vi "LVPortConvertObjectMapDataValueToVartiant.vi"(9 "Allow Variant Values (f)":bool, 10 "MatlabDataBundle":T1, 11 "Data Value":variant) -> (3 "Value":variant)   [LabVIEW 2017]
uses:
  LVPortObjectMapNamepathData.ctl
  LVPortObjectMapDataTypeEnum.ctl
  LVPortObjectMapContainerTypeEnum.ctl
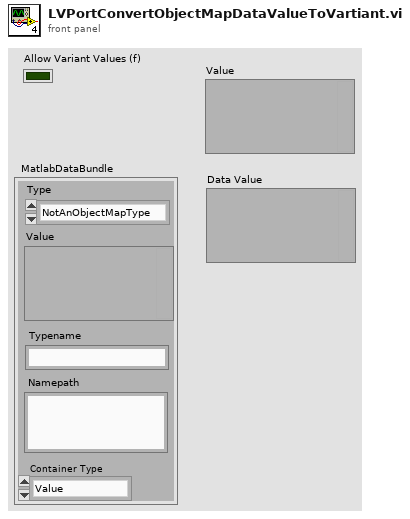
[diagram p1: front panel]
types:
  T1 = typedef "LVPortObjectMapNamepathData.ctl" = cluster{"Type":T2, "Value":variant, "Namepath":string, "Typename":string, "Container Type":T3}
  T2 = typedef "LVPortObjectMapDataTypeEnum.ctl" = enum16{"NotAnObjectMapType", "Real", "Complex", "String", "Boolean"}
  T3 = typedef "LVPortObjectMapContainerTypeEnum.ctl" = enum16{"Value", "Array", "Waveform"}
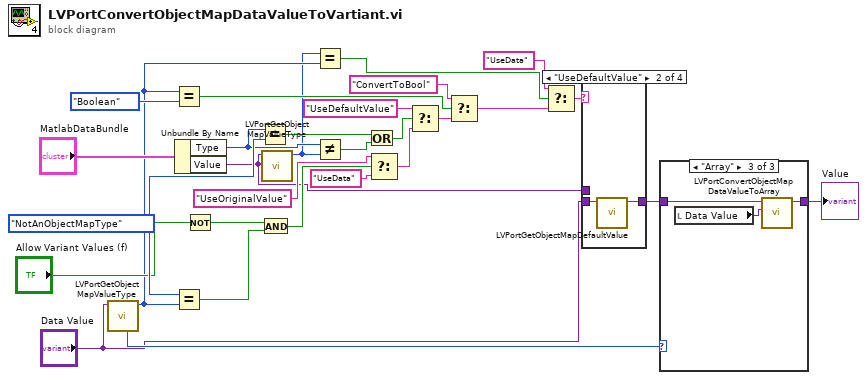
[diagram p0: block diagram]
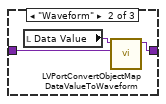
[diagram p3: hidden frame]
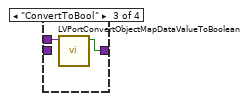
[diagram p5: hidden frame]
diagram:
  w20 = LVPortObjectMapDataTypeEnum."NotAnObjectMapType" ("MatlabType")
  n1 = call "LVPortGetObjectMapValueType.vi"("Value"="Data Value") -> ("ObjectMapType"=w10:T2, "Container Type (Labview Value type)"=w9:T3)  [unwired: 6 in, 3 out]
  n2 = Equal?(x=w10, y=LVPortObjectMapDataTypeEnum."Boolean" ("MatlabType")) -> (x = y?=w25:bool)
  n3 = Equal?(x=w20, y=w10) -> (x = y?=w17:bool)
  n4 = Unbundle By Name("MatlabDataBundle") -> ("Type"=w7:T2, "Value"=w4:variant)
  n5 = Not(x="Allow Variant Values (f)") -> (.not. x?=w19:bool)
  n6 = Equal?(x=w7, y=w20) -> (x = y?=w21:bool)
  n7 = And(x=w19, y=w17) -> (x .and. y?=w16:bool)
  n8 = call "LVPortGetObjectMapValueType.vi"("Value"=w4) -> ("ObjectMapType"=w1:T2)  [unwired: 6 in, 4 out]
  n9 = Equal?(x=w1, y=w10) -> (x = y?=w27:bool)
  n10 = Not Equal?(x=w7, y=w1) -> (x != y?=w5:bool)
  n11 = Or(x=w21, y=w5) -> (x .or. y?=w6:bool)
  n12 = Select(t="UseOriginalValue", s=w16, f="UseData") -> (s? t:f=w14:string)
  n13 = Select(t="UseDefaultValue", s=w6, f=w14) -> (s? t:f=w22:string)
  n14 = Select(t="ConvertToBool", s=w25, f=w22) -> (s? t:f=w24:string)
  n15 = Select(t="UseData", s=w27, f=w24) -> (s? t:f=w29:string)
  n16 = case shown="\"UseDefaultValue\"" w29 {
    tunnel: w4 -> [w30 _ w33 _]
    tunnel: [w30 w32 w34 w35] -> w12
    tunnel: "Data Value" -> [_ w31 _ w35]
    frame Default {
    }
    frame "UseDefaultValue" {
      n17 = call "LVPortGetObjectMapDefaultValue.vi"("From Value Type"=w31) -> ("Default Value"=w32:variant)  [unwired: 10 in]
    }
    frame "ConvertToBool" {
      n18 = call "LVPortConvertObjectMapDataValueToBoolean.vi"("Data Value"=w33) -> ("Boolean"=w34:bool)  [unwired: 10 in]
    }
    frame "UseOriginalValue" {
    }
  }
  n19 = case shown="\"Array\"" w9 {
    tunnel: w12 -> [w36 w39 w41]
    tunnel: [w36 w37 w42] -> w11
    frame Default {
    }
    frame "Waveform" {
      n20 = local read "Data Value"() -> (w38:variant)
      n21 = call "LVPortConvertObjectMapDataValueToWaveform.vi"("Numbers Vector"=w39, "Waveform"=w38) -> ("Data Value out"=w37:variant)  [unwired: 9 in]
    }
    frame "Array" {
      n22 = local read "Data Value"() -> (w40:variant)
      n23 = call "LVPortConvertObjectMapDataValueToArray.vi"("Original Value"=w40, "Data"=w41) -> ("Array"=w42:variant)  [unwired: 9 in]
    }
  }
  "Value" <- w11
